vi "Configure Waveform Characteristics.vi"   [LabVIEW 2012, in "RIGOL DG4000 Series.lvlib"]
doc: "Configure Waveform Characteristics Polymorphic VI."
uses:
  <instrlib>/RIGOL DG4000 Series/RIGOL DG4000 Series.lvlib
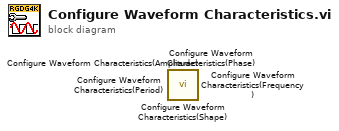
[diagram p0: block diagram]
diagram:
  n1 = call <instrlib>:"Configure Waveform Characteristics(Shape).vi"() -> ()  [unwired: 14 in, 2 out]
  n2 = call <instrlib>:"Configure Waveform Characteristics(Phase).vi"() -> ()  [unwired: 14 in, 2 out]
  n3 = call <instrlib>:"Configure Waveform Characteristics(Period).vi"() -> ()  [unwired: 14 in, 2 out]
  n4 = call <instrlib>:"Configure Waveform Characteristics(Frequency).vi"() -> ()  [unwired: 14 in, 2 out]
  n5 = call <instrlib>:"Configure Waveform Characteristics(Amplitude).vi"() -> ()  [unwired: 14 in, 2 out]
